vi "RSZVB Channel Trace Export Data With Options Extended.vi"(0 "VISA session":refnum<visa-resource-name>, 1 "Export Data (0: Complex Values)":i32(ring) items=["Complex Values", "Linear magnitude and phase", "dB-magnitude and phase"], 2 "Field Separator (0: Semicolon)":i32(ring) items=["Semicolon", "Comma", "Tabulator", "Space"], 5 "Select Channel (0: Single)":i32(ring) items=["Single", "All"], 7 "Channel (Trace) (1)":i32=1, 9 "File Name (Trc1.s1p)":string="Trc1.s1p", 11 "error in (no error)":errorcluster {"code" format="%.0x"}, 12 "Decimal Separator (0: Point)":i32(ring) items=["Point", "Comma"], 13 "Export Format (0: Unformatted)":i32(ring) items=["Unformatted", "Formatted"]) -> (4 "dup VISA session":refnum<visa-resource-name>, 15 "error out":errorcluster {"code" format="%.0x"})   [LabVIEW 2011]
doc: "This VI stores the trace data of all data traces in the specified channel to a trace file.\n\nNote(s):\n\nTraces are created using the CALCulte<Ch>:PARameter:SDEFine... command.\n\n*.s<n>p Touchstone files (<n> = 1, 2, 3, ...) are intended for a complete set of <n>-port S-parameters. Data export fails if the active channel does not contain the full set of <n>^2 traces. \n\n\nRemote-control command(s):\nMMEMory:STORe:TRACe:CHANnel <ch_number> | ALL,'<file_name>'[,UNFormatted | FORMatted, COMPlex | LINPhase | LOGPhase, POINt | COMMa, SEMicolon | COMMa | TABulator | SPACe]"
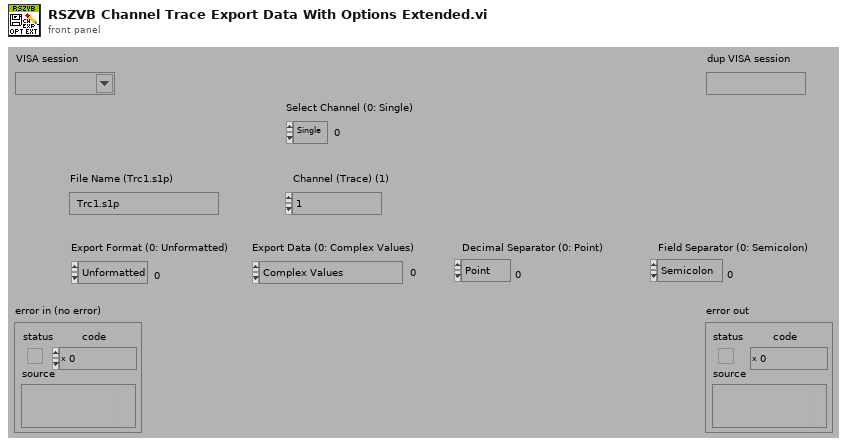
[diagram p1: front panel]
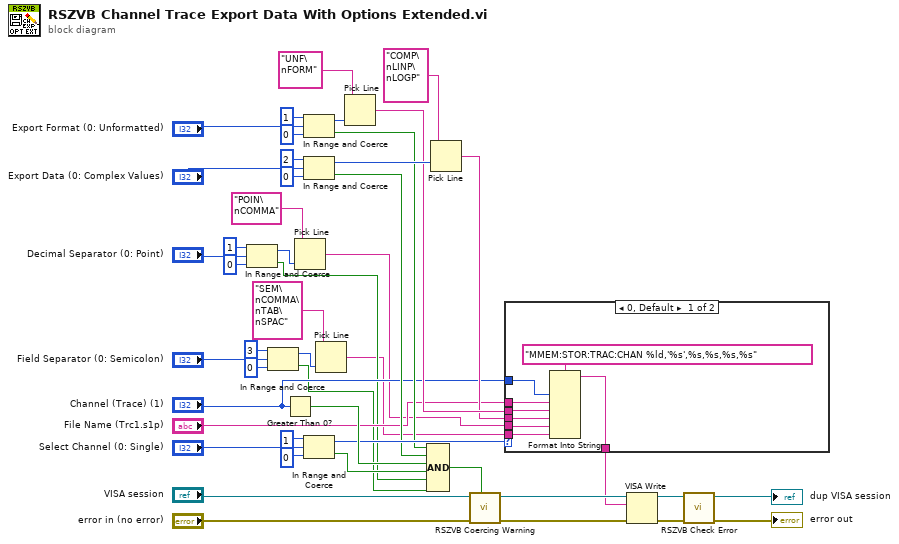
[diagram p0: block diagram]
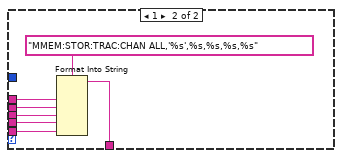
[diagram p2: hidden frame]
diagram:
  n1 = In Range and Coerce(upper limit=1, x="Decimal Separator (0: Point)", lower limit=0) -> (coerced(x)=w11:i32, In Range?=w3:bool)
  n2 = In Range and Coerce(upper limit=3, x="Field Separator (0: Semicolon)", lower limit=0) -> (coerced(x)=w7:i32, In Range?=w4:bool)
  n3 = Greater Than 0?(x="Channel (Trace) (1)") -> (x > 0?=w42:bool)
  n4 = Pick Line(multi-line string="POIN\nCOMMA", line index=w11) -> (output string=w2:string)  [unwired: 1 in]
  n5 = In Range and Coerce(upper limit=1, x="Export Format (0: Unformatted)", lower limit=0) -> (coerced(x)=w35:i32, In Range?=w27:bool)
  n6 = In Range and Coerce(upper limit=2, x="Export Data (0: Complex Values)", lower limit=0) -> (coerced(x)=w34:i32, In Range?=w26:bool)
  n7 = In Range and Coerce(upper limit=1, x="Select Channel (0: Single)", lower limit=0) -> (coerced(x)=w29:i32, In Range?=w43:bool)
  n8 = Pick Line(multi-line string="SEM\nCOMMA\nTAB\nSPAC", line index=w7) -> (output string=w1:string)  [unwired: 1 in]
  n9 = Pick Line(multi-line string="UNF\nFORM", line index=w35) -> (output string=w25:string)  [unwired: 1 in]
  n10 = Compound Arithmetic op=AND(w27, w26, w42, w43, w3, w4) -> (w46:bool)
  n11 = Pick Line(multi-line string="COMP\nLINP\nLOGP", line index=w34) -> (output string=w24:string)  [unwired: 1 in]
  n12 = call "RSZVB Coercing Warning.vi"("In Range?"=w46, "error in (no error)"="error in (no error)", "VISA session"="VISA session") -> ("error out"=w30:errorcluster, "dup VISA session"=w33:refnum<visa-resource-name>)  [unwired: 7 in]
  n13 = case shown="0, Default" w29 {
    tunnel: [w54 w61] -> w28
    tunnel: "Channel (Trace) (1)" -> [w52 _]
    tunnel: "File Name (Trc1.s1p)" -> [w51 w59]
    tunnel: w25 -> [w50 w58]
    tunnel: w24 -> [w49 w57]
    tunnel: w2 -> [w48 w56]
    tunnel: w1 -> [w47 w55]
    frame 0, Default {
      n14 = Format Into String(format string="MMEM:STOR:TRAC:CHAN %ld,'%s',%s,%s,%s,%s", w52, w51, w50, w49, w48, w47) -> (resulting string=w54:string)  [unwired: 2 in, 1 out]
    }
    frame 1 {
      n15 = Format Into String(format string="MMEM:STOR:TRAC:CHAN ALL,'%s',%s,%s,%s,%s", w59, w58, w57, w56, w55) -> (resulting string=w61:string)  [unwired: 2 in, 1 out]
    }
  }
  n16 = VISA Write(VISA resource name=w33, write buffer=w28, error in (no error)=w30) -> (VISA resource name out=w32:refnum<visa-resource-name>, error out=w31:errorcluster)  [unwired: 1 out]
  n17 = call "RSZVB Check Error.vi"("error in (no error)"=w31, "VISA session"=w32) -> ("error out"=→"error out":errorcluster, "dup VISA session"=→"dup VISA session":refnum<visa-resource-name>)  [unwired: 8 in]
